vi "Read Auto Refresh.vi"(8 "error in (no error)":errorcluster, 11 "Connection Data In":T3) -> (0 "error out":errorcluster, 1 "Adquisition Data Out":T2, 3 "Connection Data Out":T3)   [LabVIEW 2014, in "MSX-E3701_dll.lvlib"]
doc: "Inicia la adquisición de datos en modo AutoRefresh. Al mismo tiempo lee el estado de las I/O."
uses:
  MSX-E3701_dll.lvlib
  Typedef/Connection Data.ctl
  E:/Repositorio Magnis/INF002/v0/Modules/HAL/Drivers/Sync/ADDI-DATA MSX-E3701/API/MX370x.dll
  MX370x.dll
  E:/Repositorio Magnis/INF002/v0/Modules/HAL/Drivers/Sync/ADDI-DATA MSX-E3701/API/MXCommon.dll
  MXCommon.dll
  Typedef/Adquisition Data.ctl
  Typedef/Config Data.ctl
panel:
  in  "Config Data":T1
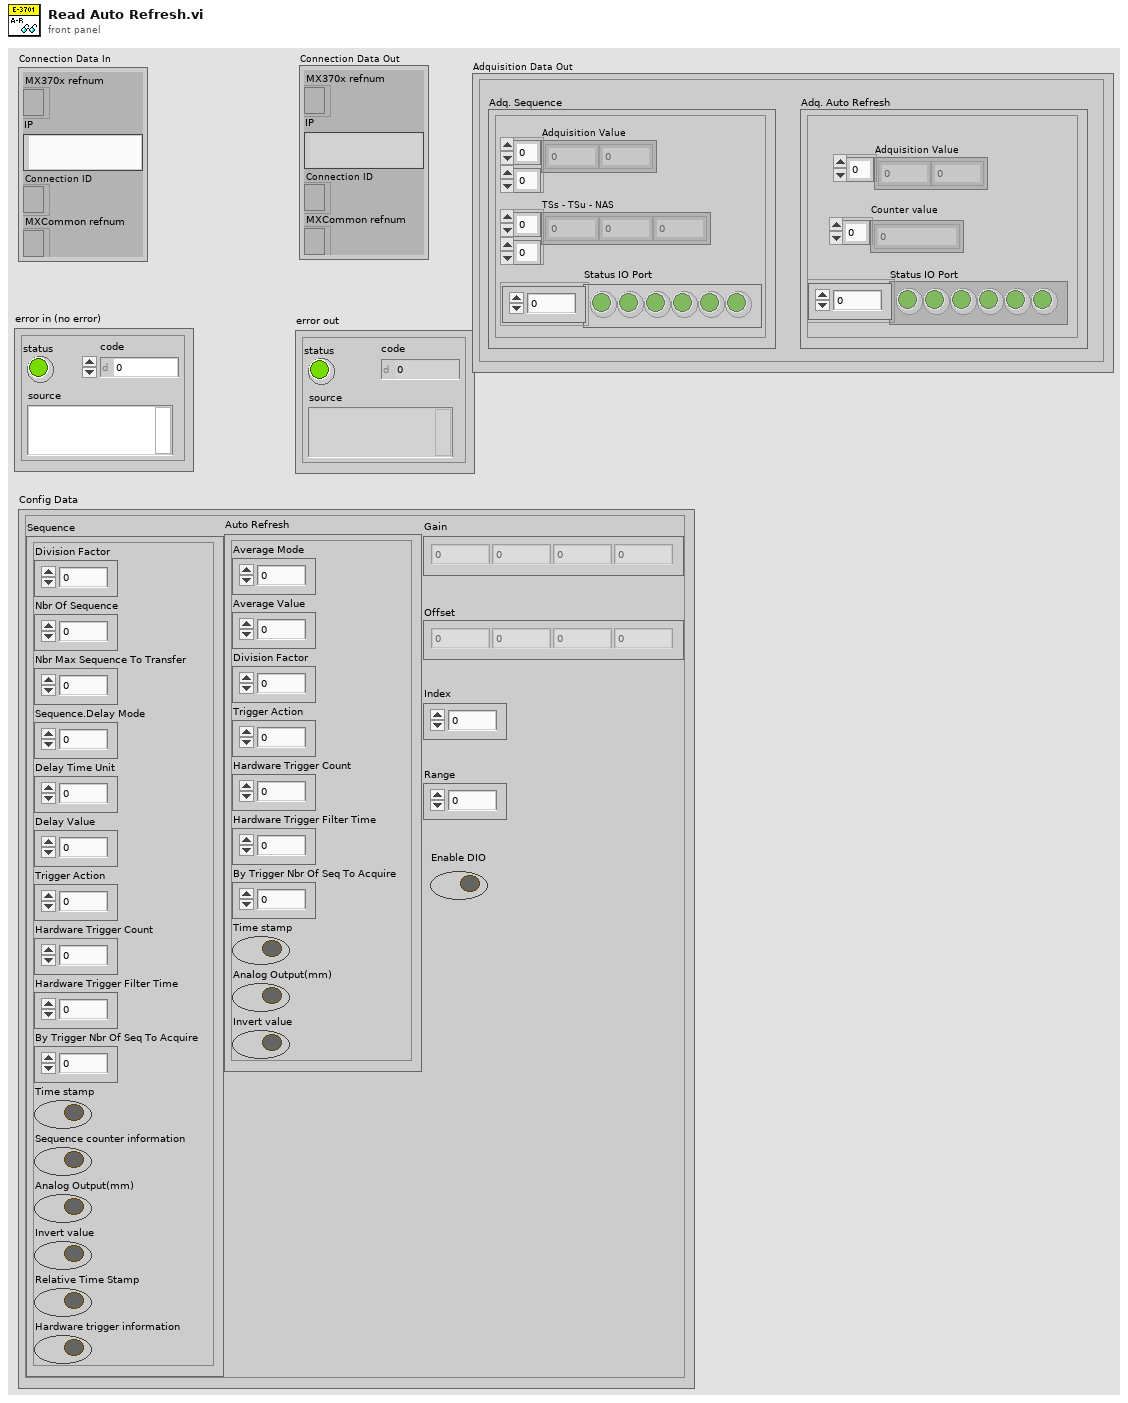
[diagram p1: front panel]
types:
  T1 = typedef "MSX-E3701_dll.lvlib/Config Data.ctl" = cluster{"Auto Refresh":cluster{"Average Mode":u64, "Average Value":u64, "Division Factor":u64, "Trigger Action":u64, "Hardware Trigger Count":u64, "Hardware Trigger Filter Time":u64, "By Trigger Nbr Of Seq To Acquire":u64, "Time stamp":bool, "Analog Output(mm)":bool, "Invert value":bool}, "Gain":sgl[], "Offset":sgl[], "Index":u64, "Range":sgl, "Sequence":cluster{"Division Factor":u64, "Nbr Of Sequence":u64, "Nbr Max Sequence To Transfer":u64, "Sequence.Delay Mode":u64, "Delay Time Unit":u64, "Delay Value":u64, "Trigger Action":u64, "Hardware Trigger Count":u64, "Hardware Trigger Filter Time":u64, "By Trigger Nbr Of Seq To Acquire":u64, "Time stamp":bool, "Sequence counter information":bool, "Analog Output(mm)":bool, "Invert value":bool, "Relative Time Stamp":bool, "Hardware trigger information":bool}, "Enable DIO":bool}
  T2 = typedef "MSX-E3701_dll.lvlib/Adquisition Data.ctl" = cluster{"Adq. Sequence":cluster{"TSs - TSu - NAS":u64[][], "Adquisition Value":u32[][], "Status IO Port":bool[]}, "Adq. Auto Refresh":cluster{"Adquisition Value":u64[], "Status IO Port":bool[], "Counter value":u64[]}}
  T3 = typedef "MSX-E3701_dll.lvlib/Connection Data.ctl" = cluster{"MX370x refnum":refnum<k24>, "IP":string, "Connection ID ":refnum<k5>, "MXCommon refnum":refnum<k24>}
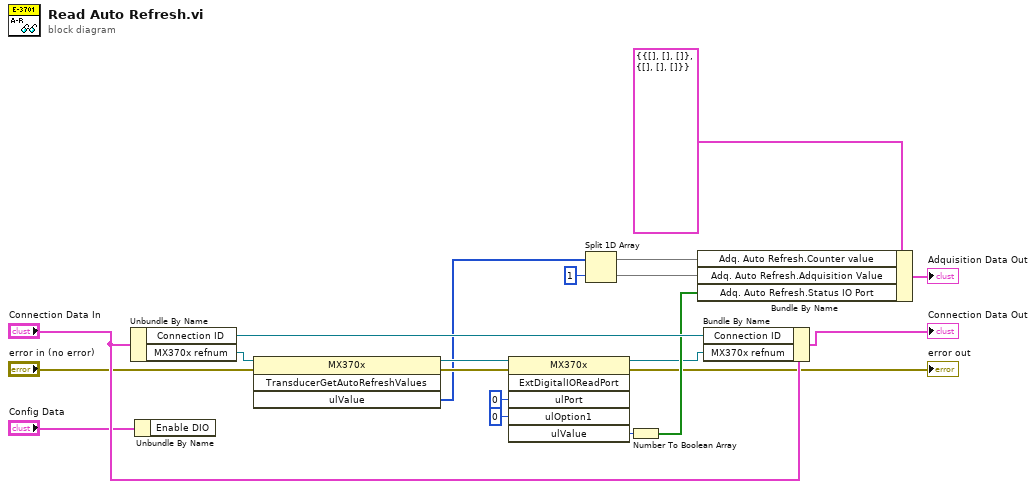
[diagram p0: block diagram]
diagram:
  n1 = Unbundle By Name("Connection Data In") -> ("Connection ID"=w16:refnum<k5>, "MX370x refnum"=w12:refnum<k24>)
  n2 = Unbundle By Name("Config Data") -> ()  [unwired: 1 out]
  n3 = invoke class="MX370x" method="TransducerGetAutoRefreshValues"(reference=w12, error in="error in (no error)") -> (reference out=w7:refnum<k24>, error out=w10:errorcluster, "ulValue"=w6:u64[])  [unwired: 2 in, 1 out]
  n4 = invoke class="MX370x" method="ExtDigitalIOReadPort"(reference=w7, error in=w10, "ulPort"=u64 0, "ulOption1"=u64 0) -> (reference out=w8:refnum<k24>, error out=→"error out":errorcluster, "ulValue"=w3:u64)  [unwired: 2 in, 3 out]
  n5 = Split 1D Array(array=w6, index=1) -> (first subarray=w13:u64[], second subarray=w5:u64[])
  n6 = Number To Boolean Array(number=w3) -> (Boolean array=w14:bool[])
  n7 = Bundle By Name(cluster=T2 {"Adq. Sequence"={"TSs - TSu - NAS"=[], "Adquisition Value"=[], "Status IO Port"=[]}, "Adq. Auto Refresh"={"Adquisition Value"=[], "Status IO Port"=[], "Counter value"=[]}} ("Adquisition Data In"), "Adq. Auto Refresh.Counter value"=w13, "Adq. Auto Refresh.Adquisition Value"=w5, "Adq. Auto Refresh.Status IO Port"=w14) -> (→"Adquisition Data Out":T2)
  n8 = Bundle By Name(cluster="Connection Data In", "Connection ID"=w16, "MX370x refnum"=w8) -> (→"Connection Data Out":T3)
